vi "Get Recoverable Network Streams Errors.vi"() -> (3 "recoverable network streams errors":i32[](array[numeric]) caption="可恢复的网络流错误")   [LabVIEW 2015]
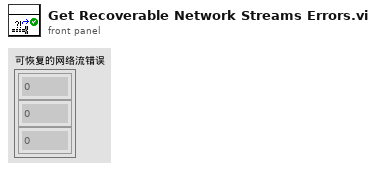
[diagram p1: front panel]
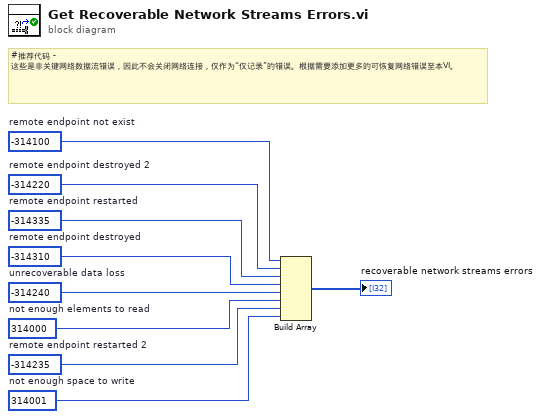
[diagram p0: block diagram]
diagram:
  w1 = -314100  # remote endpoint not exist
  w2 = -314220  # remote endpoint destroyed 2
  w4 = 314001  # not enough space to write
  w6 = 314000  # not enough elements to read
  w5 = -314235  # remote endpoint restarted 2
  w7 = -314240  # unrecoverable data loss
  w8 = -314310  # remote endpoint destroyed
  w9 = -314335  # remote endpoint restarted
  # "#推荐代码 - 这些是非关键网络数据流错误，因此不会关闭网络连接，仅作为“仅记录”的错误。根据需要添加更多的可恢复网络错误至本VI。"
  n1 = Build Array(w1, w2, w9, w8, w7, w6, w5, w4) -> (→"recoverable network streams errors":i32[])
